vi "close_refs.vi"(8 "error in":errorcluster, 11 "Refs[]  In":refnum<vi>[](array[refnum])) -> (0 "error out":errorcluster)   [LabVIEW 2018]
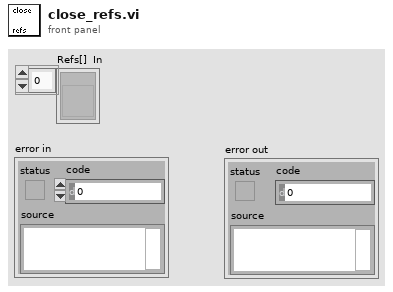
[diagram p1: front panel]
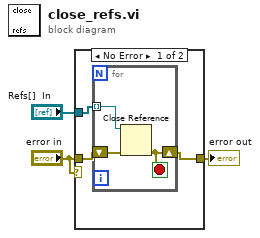
[diagram p0: block diagram]
diagram:
  n1 = case shown="No Error" "error in" {
    tunnel: [w6 w10] -> w3
    tunnel: "error in" -> [w5 w10]
    tunnel: "Refs[]  In" -> [w4 _]
    frame No Error {
      n2 = for {
        tunnel: w4 -> [w9] mode=indexing
        shift-right: [w7] -> w6
        shift-left: w5 -> [w8]
        stop <- w7 stop-if-true
        n3 = Close Reference(reference=w9, error in (no error)=w8) -> (error out=w7:errorcluster)
      }
    }
    frame Error {
    }
  }
  "error out" <- w3
